vi "get tree refnum.vi"(8 "Error In":errorcluster, 9 "Do for all Child Sections?":bool=TRUE caption="Do for all Child Sections? (T)", 10 "Open?":bool caption="Open? (F)", 11 "Item Ref in":T1 format="%.0x") -> (0 "Error Out":errorcluster, 3 "Item Ref out":T1 format="%.0x")   [LabVIEW 2018, in "CAN Gateway System Explorer.lvlib"]
uses:
  CAN Gateway System Explorer.lvlib
  <vilib>/NI Veristand/Custom Device API/Custom Device Item Ref.ctl
  <vilib>/Utility/traverseref.llb/TRef TravTarget.ctl
  <vilib>/Utility/traverseref.llb/VI Scripting - Traverse.lvlib
  <vilib>/NI Veristand/Custom Device API/Custom Device API.lvlib
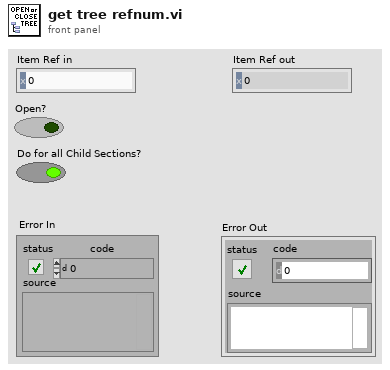
[diagram p1: front panel]
types:
  T1 = typedef "Custom Device API.lvlib/Custom Device Item Ref.ctl" = u64
  T2 = typedef "TRef TravTarget.ctl" = enum16{"FP", "BD", "Other"}
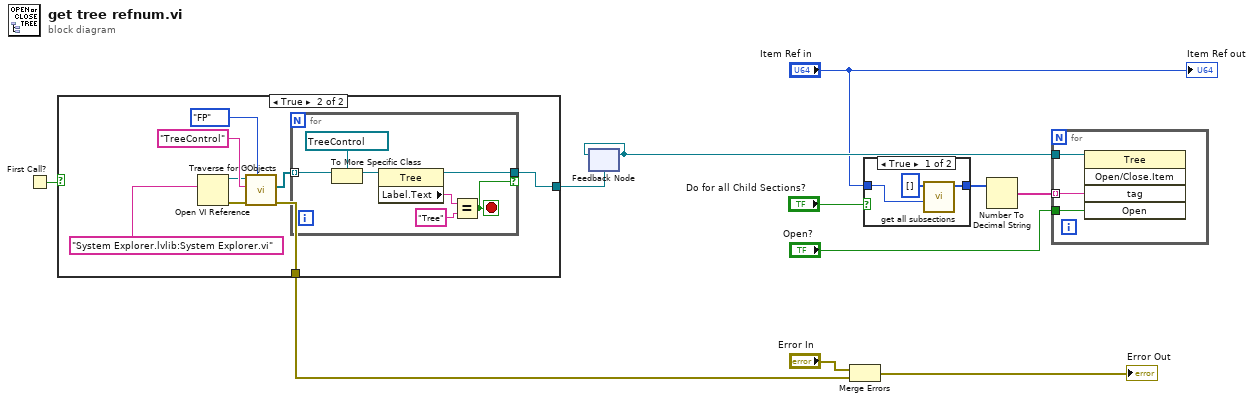
[diagram p0: block diagram]
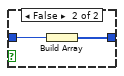
[diagram p2: hidden frame]
diagram:
  n1 = First Call?() -> (First Call?: T/F=w9:bool)
  n2 = case shown="True" w9 {
    tunnel: [_ w16] -> w11
    tunnel: [_ w13] -> w8
    frame False {
    }
    frame True {
      n3 = Open VI Reference(vi path="System Explorer.lvlib:System Explorer.vi" ("Class Name")) -> (vi reference=w15:refnum<vi>, error out=w14:errorcluster)  [unwired: 5 in]
      n4 = call <vilib>:"Traverse for GObjects.vi"("Traverse Target"=TRef_TravTarget."FP", "error in (no error)"=w14, "Class Name"="TreeControl", "VI Refnum"=w15) -> ("error out"=w13:errorcluster, "References"=w17:refnum<vi>[])  [unwired: 4 in, 2 out]
      n5 = for {
        tunnel: w17 -> [w26] mode=indexing
        tunnel: [w21] -> w16 if=w20
        stop <- w20 stop-if-true
        n6 = To More Specific Class(target class=refnum<vi> refnum ("Tree"), reference=w26) -> (specific class reference=w25:refnum<vi>)  [unwired: 1 in, 1 out]
        n7 = property class="Tree"(reference=w25) -> (reference out=w21:refnum<vi>, "Label.Text"=w22:string)  [unwired: 1 in, 1 out]
        n8 = Equal?(x=w22, y="Tree" ("Class Name")) -> (x = y?=w20:bool)
      }
    }
  }
  n9 = feedback #1(w11) -> (w10:refnum<vi>)
  n10 = feedback-in #1(w10) -> ()
  n11 = Merge Errors("Error In", w8) -> (→"Error Out":errorcluster)
  n12 = case shown="True" "Do for all Child Sections?" {
    tunnel: "Item Ref in" -> [w29 w31]
    tunnel: [w28 w30] -> w3
    frame True {
      n13 = call "get all subsections.vi"("Item Ref in"=w29, "Child Sections In"=T1[] []) -> ("Child Sections Out"=w28:T1[])  [unwired: 8 in, 1 out]
    }
    frame False {
      n14 = Build Array(w31) -> (w30:T1[])
    }
  }
  n15 = Number To Decimal String(number=w3) -> (decimal integer string=w2:string[])  [unwired: 1 in]
  n16 = for {
    tunnel: "Open?" -> [w34]
    tunnel: w10 -> [w33]
    tunnel: w2 -> [w32] mode=indexing
    n17 = invoke class="Tree" method="Open/Close.Item"(reference=w33, "tag"=w32, "Open"=w34) -> ()  [unwired: 2 in, 5 out]
  }
  "Item Ref out" <- "Item Ref in"
